vi "Mark Target Centers.vi"(1 "Processed Image":T2(plugin-control), 2 "Target Info":T1(array[cluster])) -> (0 "Image Out":T2(plugin-control))   [LabVIEW 2011]
doc: "This SubVI is used to mark the target's centers in their appropriate order.\n\nThe order is left-to-right: the left target on the array on your left is Target no. 1, and the right one is 4."
panel:
  # "This SubVI is used to mark the target's centers in their appropriate order.\nThe order is left-to-right: the left target on the array on your left is Target no. 1, and the right one is 4."
  # "1"
  # "2"
  # "3"
  # "4"
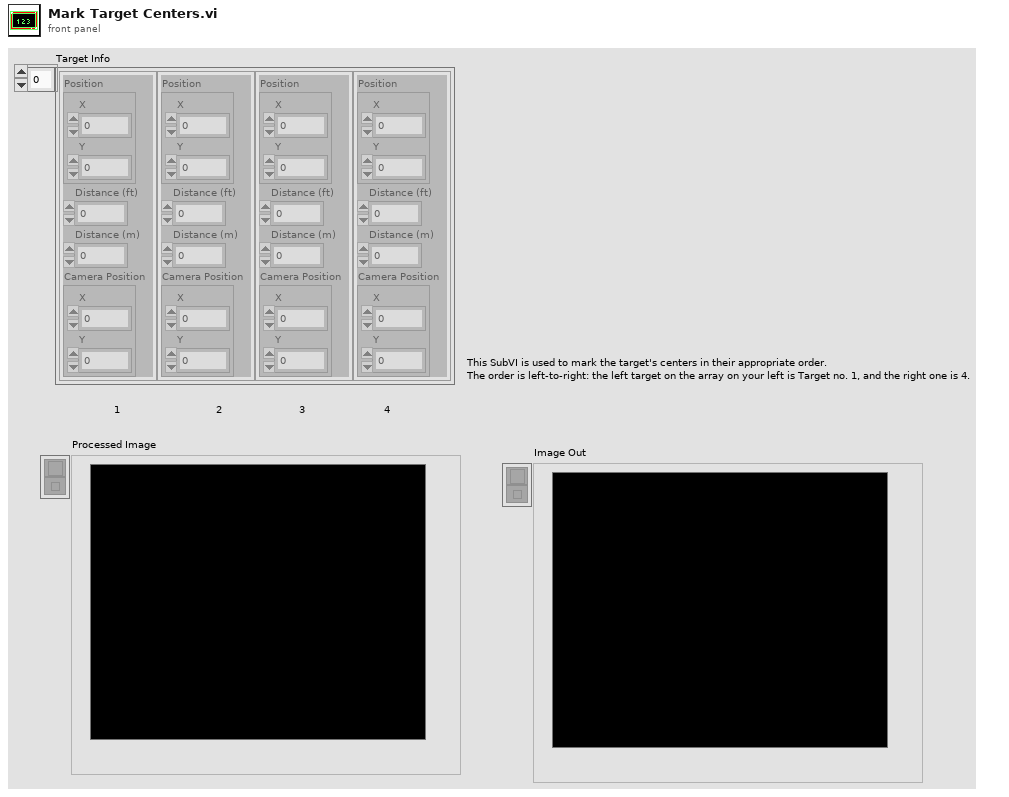
[diagram p1: front panel]
types:
  T1 = cluster{"Position":cluster{"X":dbl, "Y":dbl}, "Distance (ft)":dbl, "Distance (m)":dbl, "Camera Position":cluster{"X":dbl, "Y":dbl}}[]
  T2 = typedef "IMAQ Image.ctl" = refnum<image>
  T3 = cluster{"Position":cluster{"X":dbl, "Y":dbl}, "Distance (ft)":dbl, "Distance (m)":dbl, "Camera Position":cluster{"X":dbl, "Y":dbl}}
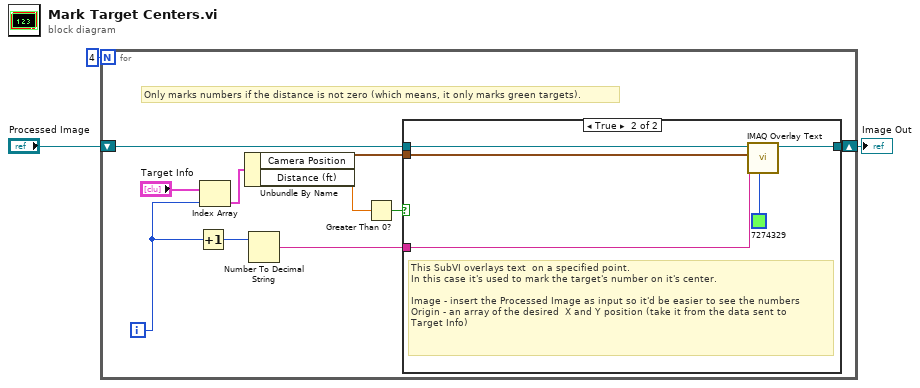
[diagram p0: block diagram]
diagram:
  n1 = for {
    N: 4 -> [_]
    shift-right: [w9] -> w1
    shift-left: "Processed Image" -> [w8]
    i -> [w13]
    # "Only marks numbers if the distance is not zero (which means, it only marks green targets)."
    n2 = Increment(x=w13) -> (x+1=w12:i32)
    n3 = Index Array(array="Target Info", index=w13) -> (element=w10:T3)
    n4 = Unbundle By Name(w10) -> ("Camera Position"=w6:cluster{"X":dbl, "Y":dbl}, "Distance (ft)"=w4:dbl)
    n5 = Number To Decimal String(number=w12) -> (decimal integer string=w11:string)  [unwired: 1 in]
    n6 = Greater Than 0?(x=w4) -> (x > 0?=w5:bool)
    n7 = case shown="True" w5 {
      tunnel: w11 -> [_ w18]
      tunnel: w6 -> [_ w17]
      tunnel: [w14 w16] -> w9
      tunnel: w8 -> [w14 w15]
      frame False {
      }
      frame True {
        # "This SubVI overlays text  on a specified point.\nIn this case it's used to mark the target's number on it's center.\n\nImage - insert the Processed Image as input so it'd be easier to see the numbers\nOrigin - an array of the desired  X and Y position (take it from the data sent to\nTarget Info)"
        n8 = call "IMAQ Overlay Text"("Text Color (black)"=u32 7274329 ("Color"), "String"=w18, "Origin"=w17, "Image"=w15) -> ("Image Out"=w16:T2)  [unwired: 6 in, 1 out]
      }
    }
  }
  "Image Out" <- w1
